vi "Target.vi"() -> ()   [LabVIEW 2025]
panel:
  out "Array 3":bool[](array[boolean])
  out "Array 2":i32[](array[numeric])
  out "Array":bool[](array[boolean])
  out "C":fxp<+/-,32,16>[](array[numeric])
  out "Cycle Count":i32
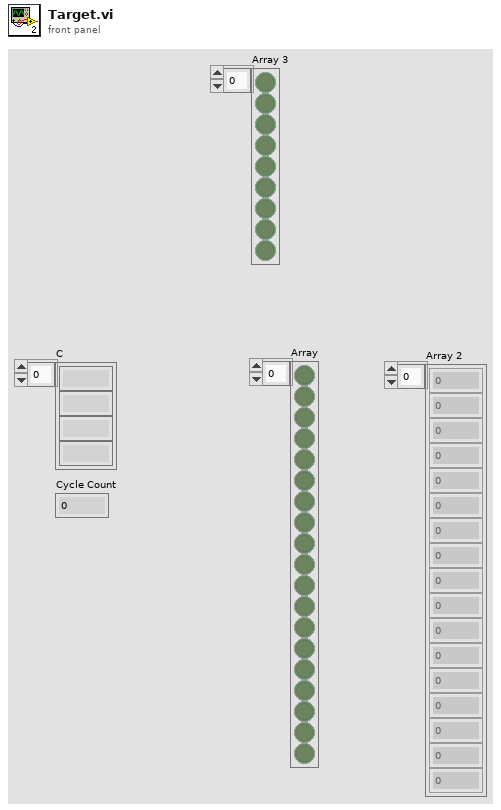
[diagram p1: front panel]
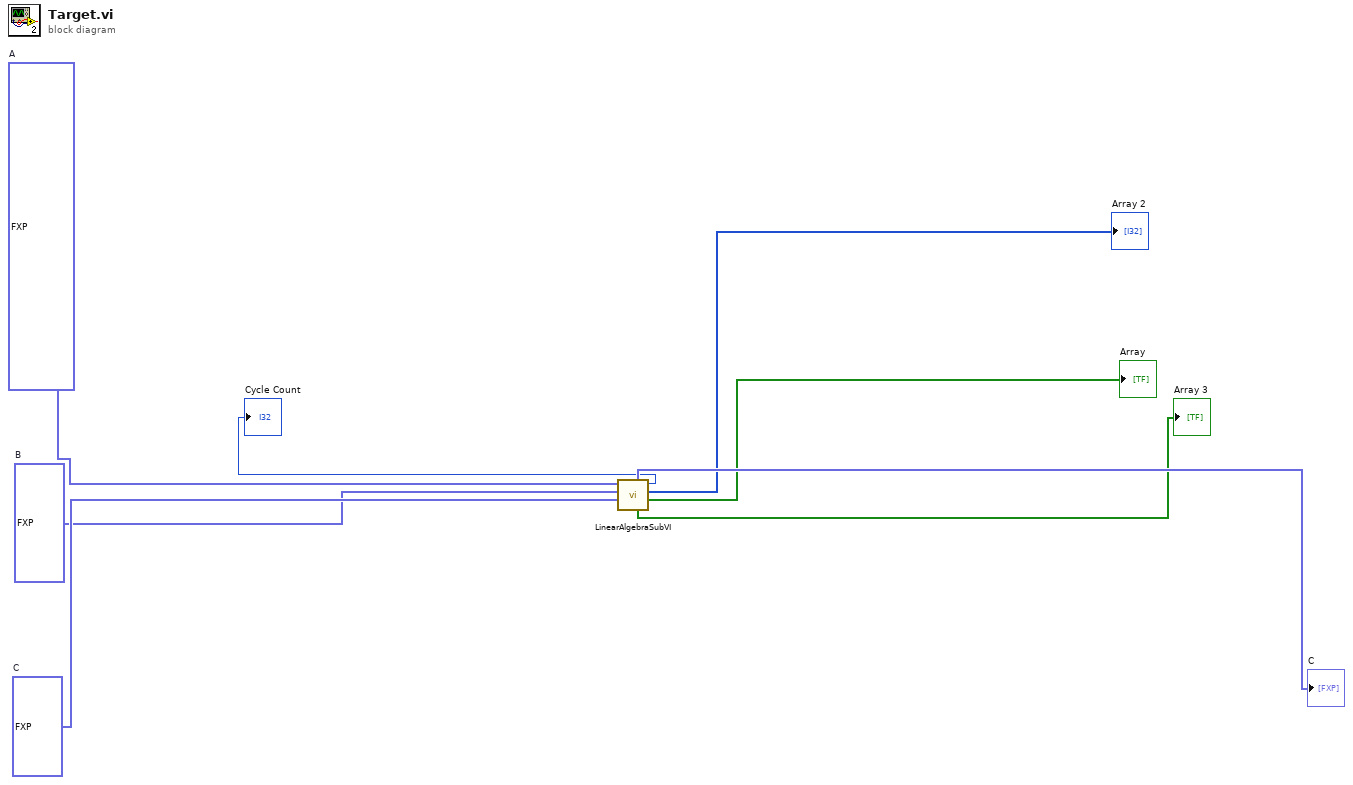
[diagram p0: block diagram]
diagram:
  w6 = fxp<+/-,32,16>[] [1.0, 2.0, 3.0, 4.0, 5.0, 6.0, 7.0, 8.0, 9.0, 10.0, 11.0, 12.0, 13.0, 14.0, 15.0, 16.0]  # A
  w7 = fxp<+/-,32,16>[] [1.0, 2.0, 3.0, 4.0]  # B
  w8 = fxp<+/-,32,16>[] [0.0, 0.0, 0.0, 0.0]  # C
  n1 = call "LinearAlgebraSubVI.vi"("C in"=w8, "B"=w7, "A"=w6) -> ("Array"=→"Array":bool[], "Array 2"=→"Array 2":i32[], "Cycle Count"=→"Cycle Count":i32, "Array 3"=→"Array 3":bool[], "C out"=→"C":fxp<+/-,32,16>[])  [unwired: 4 in]
